vi "ad discrete out.vi"(7 "data":u32, 8 "error in (no error)":errorcluster, 9 "range":i32, 10 "cha":i32, 11 "adh":i32) -> (0 "error out":errorcluster, 3 "function return":i32)   [LabVIEW 2021, in "libad4.lvlib"]
doc: "ad_discrete_out (int32_t adh, int32_t cha, int32_t range, uint32_t data);\n\nSets an output. Note that if the DAQ does not support setting output ranges via software, then the value passed to the VI must match the one expected by the device.s"
uses:
  <userlib>/libad4/libad4.lvlib
  <userlib>/libad4/libad4.dll
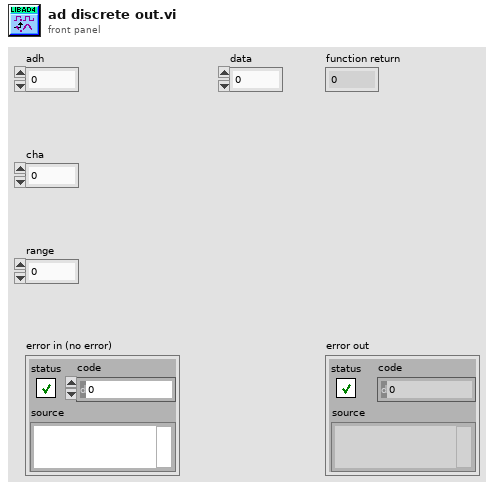
[diagram p1: front panel]
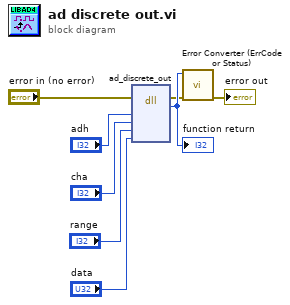
[diagram p0: block diagram]
diagram:
  n1 = dll-call lib="C:/Program Files/National Instruments/LabVIEW 2021/user.lib/libad4/libad4.*" fn="ad_discrete_out"(error in="error in (no error)", "adh"="adh", "cha"="cha", "range"="range", "data"="data") -> (error out=w2:errorcluster, "return type"=w8:i32)  [unwired: 6 in, 1 out]
  "function return" <- w8
  n2 = call <userlib>:"Error Converter (ErrCode or Status).vi"("error in (no error)"=w2, "error code"=w8) -> ("error out"=→"error out":errorcluster)  [unwired: 9 in]
